vi "Template.vi"() -> ()   [LabVIEW 2018]
uses:
  <vilib>/Instr/_visa.llb/VISA Configure Serial Port (Instr).vi
panel:
  in  "stop":bool
  out "Response":enum16{"Push", "Pull", "Pause"}(ring)
  out "FakeError":bool
  out "Data":dbl[](array[numeric])
  in  "Do Command":bool
  in  "Command":enum16{"Push", "Pull", "Pause"}(ring)
  in  "VISA resource name":refnum<visa-resource-name>
  # "Try to organize your front panel in an organized way.\nThe cleaner it is, the easier it is for others (and you) to run your vi."
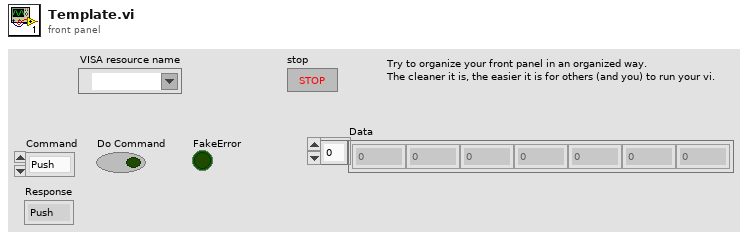
[diagram p1: front panel]
types:
  T1 = enum16{"open", "open or create", "create or replace", "create", "open (read-only)"}
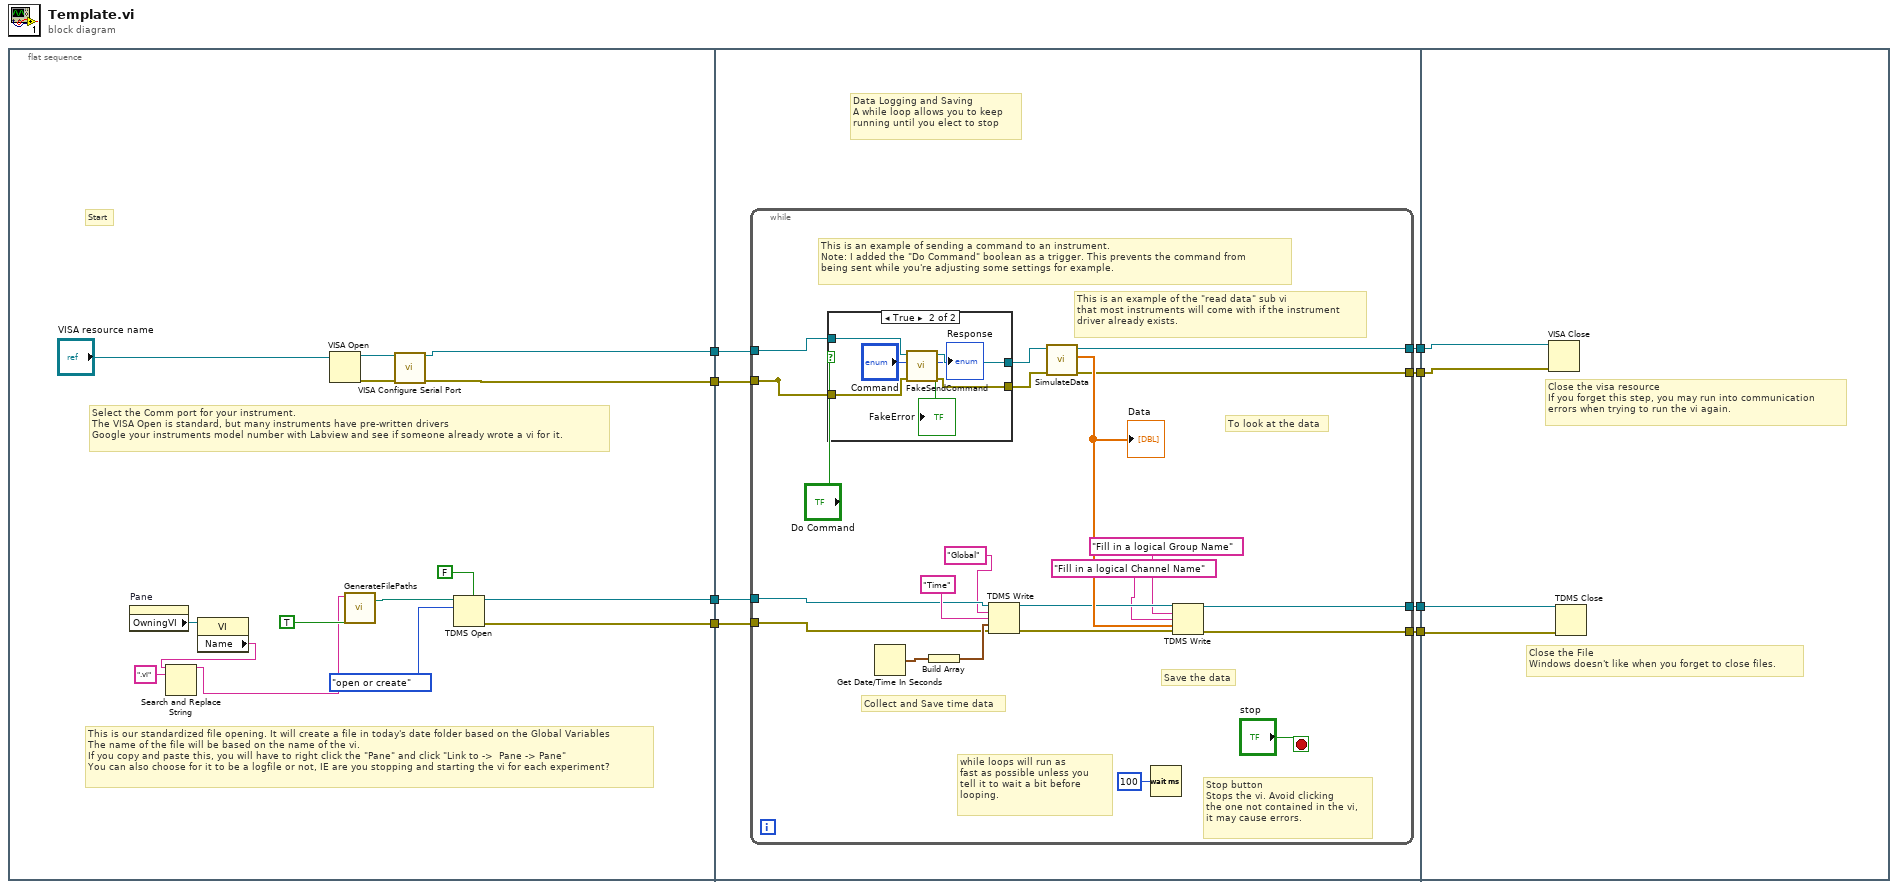
[diagram p0: block diagram]
diagram:
  n1 = flat-sequence {
    tunnel: [w14] -> w8
    tunnel: [w13] -> w7
    tunnel: [w12] -> w6
    tunnel: [w11] -> w5
    tunnel: w8 -> [w31]
    tunnel: w7 -> [w30]
    tunnel: w6 -> [w29]
    tunnel: w5 -> [w28]
    tunnel: [w27] -> w4
    tunnel: [w26] -> w3
    tunnel: [w25] -> w2
    tunnel: [w24] -> w1
    tunnel: w4 -> [w66]
    tunnel: w3 -> [w65]
    tunnel: w2 -> [w64]
    tunnel: w1 -> [w63]
    frame #0 {
      # "This is our standardized file opening. It will create a file in today's date folder based on the Global Variables\nThe name of the file will be based on the name of the vi. \nIf you copy and paste this, you will have to right click the \"Pane\" and click \"Link to ->  Pane -> Pane\"\nYou can also choose for it to be a logfile or not, IE are you stopping and starting the vi for each experiment?"
      # "Select the Comm port for your instrument.\nThe VISA Open is standard, but many instruments have pre-written drivers\nGoogle your instruments model number with Labview and see if someone already wrote a vi for it."
      # "Start"
      n2 = property on="Pane" class="Pane"() -> ("OwningVI"=w20:refnum<vi>)  [unwired: 2 in, 2 out]
      n3 = property class="VI"(reference=w20) -> ("Name"=w17:string)  [unwired: 1 in, 2 out]
      n4 = Search and Replace String(input string=w17, search string=".vi") -> (result string=w18:string)  [unwired: 6 in, 3 out]
      n5 = VISA Open(VISA resource name="VISA resource name") -> (VISA resource name=w10:refnum<visa-resource-name>, error out=w9:errorcluster)  [unwired: 4 in]
      n6 = call "GenerateFilePaths.vi"("Logfile? (F)"=TRUE, "Device Name"=w18) -> ("Path"=w22:path)  [unwired: 3 in]
      n7 = call-poly "VISA Configure Serial Port"("VISA resource name"=w10, "error in (no error)"=w9) -> ("VISA resource name out"=w14:refnum<visa-resource-name>, "error out"=w13:errorcluster)  [unwired: 12 in]
      n8 = TDMS Open(5:FALSE ("create index file? (T)"), 10:T1."open or create" ("operation (0:open)"), 11:w22) -> (0:w11:errorcluster, 3:w12:refnum<k34>)  [unwired: 4 in]
    }
    frame #1 {
      # "Data Logging and Saving\nA while loop allows you to keep\nrunning until you elect to stop"
      n9 = while {
        tunnel: w31 -> [w42]
        tunnel: [w39] -> _
        tunnel: w30 -> [w39]
        tunnel: w29 -> [w50]
        tunnel: w28 -> [w49]
        tunnel: [w44] -> w27
        tunnel: [w43] -> w26
        tunnel: [w37] -> w25
        tunnel: [w36] -> w24
        stop <- "stop" stop-if-true
        # "Stop button\nStops the vi. Avoid clicking\nthe one not contained in the vi,\nit may cause errors."
        # "while loops will run as\nfast as possible unless you\ntell it to wait a bit before \nlooping."
        # "Save the data"
        # "Collect and Save time data"
        # "To look at the data"
        # "This is an example of the \"read data\" sub vi\nthat most instruments will come with if the instrument\ndriver already exists."
        # "This is an example of sending a command to an instrument.\nNote: I added the \"Do Command\" boolean as a trigger. This prevents the command from\nbeing sent while you're adjusting some settings for example."
        n10 = case shown="True" "Do Command" {
          tunnel: w42 -> [w55 w61]
          tunnel: [w55 w60] -> w41
          tunnel: [w54 w59] -> w40
          tunnel: w39 -> [w54 w58]
          frame False {
          }
          frame True {
            n11 = call "FakeSendCommand.vi"("error in (no error)"=w58, "Enum"="Command", "VISA resource name"=w61) -> ("error out"=w59:errorcluster, "FakeError"=→"FakeError":bool, "Response"=→"Response":enum16{"Push", "Pull", "Pause"}, "VISA resource name out"=w60:refnum<visa-resource-name>)  [unwired: 5 in]
          }
        }
        n12 = Get Date/Time In Seconds() -> (seconds since 1Jan1904=w53:timestamp)
        n13 = Build Array(w53) -> (w52:timestamp[])
        n14 = TDMS Write(0:w50, 5:"Global" ("group name in (Untitled)"), 7:"Time", 9:w52, 11:w49) -> (4:w46:refnum<k34>, 15:w45:errorcluster)  [unwired: 1 in, 2 out]
        n15 = call "SimulateData.vi"("error in (no error)"=w40, "VISA resource name"=w41) -> ("error out"=w43:errorcluster, "Data"=w47:dbl[], "VISA resource name out"=w44:refnum<visa-resource-name>)  [unwired: 7 in]
        "Data" <- w47
        n16 = Wait (ms)(milliseconds to wait=u32 100) -> ()  [unwired: 1 out]
        n17 = TDMS Write(0:w46, 5:"Fill in a logical Group Name" ("group name in (Untitled)"), 7:"Fill in a logical Channel Name" ("group name in (Untitled)"), 9:w47, 11:w45) -> (4:w37:refnum<k34>, 15:w36:errorcluster)  [unwired: 1 in, 2 out]
      }
    }
    frame #2 {
      # "Close the visa resource\nIf you forget this step, you may run into communication\nerrors when trying to run the vi again."
      # "Close the File\nWindows doesn't like when you forget to close files."
      n18 = VISA Close(VISA resource name=w66, error in (no error)=w65) -> ()  [unwired: 1 out]
      n19 = TDMS Close(8:w63, 11:w64) -> ()  [unwired: 2 out]
    }
  }
